vi "Maint_u_2.vi"() -> ()   [LabVIEW 2011]
uses:
  Globals/Global VI.vi
panel:
  in  "Process Stop Button":bool
  out "Boolean":bool
  # "Maintenance"
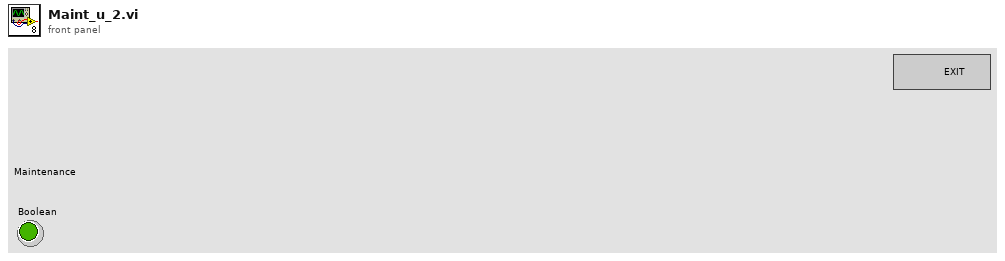
[diagram p1: front panel]
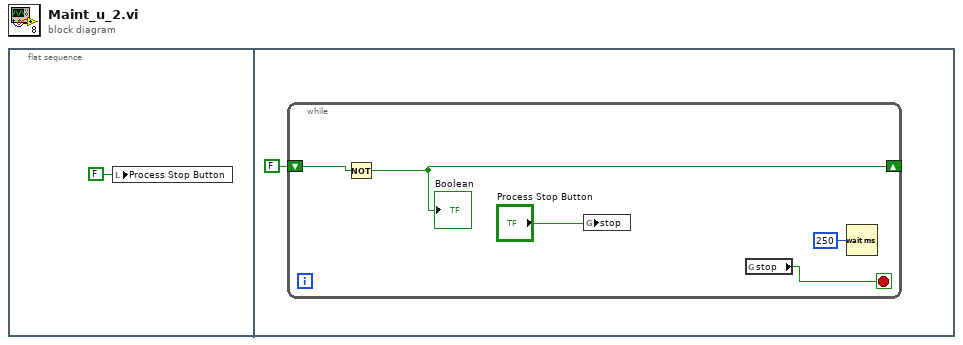
[diagram p0: block diagram]
diagram:
  n1 = flat-sequence {
    frame #0 {
      n2 = local write "Process Stop Button"(FALSE ("Process Stop Button")) -> ()
    }
    frame #1 {
      n3 = while {
        shift-right: [w4] -> _
        shift-left: FALSE -> [w5]
        stop <- w6 stop-if-true
        n4 = Not(x=w5) -> (.not. x?=w4:bool)
        "Boolean" <- w4
        n5 = global write "Global VI.vi" "stop"("Process Stop Button") -> ()
        n6 = global read "Global VI.vi" "stop"() -> (w6:bool)
        n7 = Wait (ms)(milliseconds to wait=u32 250) -> ()  [unwired: 1 out]
      }
    }
  }
